vi "WriteToLogFile.vi"(7 "Prepend timestamp":bool, 8 "error in (no error)":errorcluster, 10 "Log entry":string, 11 "Byte Stream File in":refnum<file>) -> (0 "error out":errorcluster, 3 "refnum out":refnum<file>)   [LabVIEW 2019, in "SolutionBuilder.lvlib"]
uses:
  SolutionBuilder/SolutionBuilder.lvlib
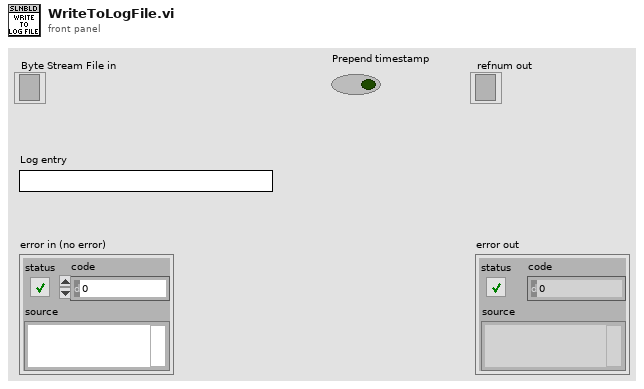
[diagram p1: front panel]
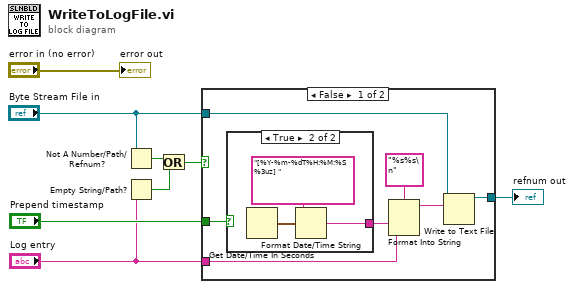
[diagram p0: block diagram]
diagram:
  n1 = Not A Number/Path/Refnum?(number/path/refnum="Byte Stream File in") -> (NaN/Path/Refnum?=w6:bool)
  n2 = Empty String/Path?(string/path="Log entry") -> (empty?=w4:bool)
  n3 = Or(x=w6, y=w4) -> (x .or. y?=w5:bool)
  n4 = case shown="False" w5 {
    tunnel: "Log entry" -> [w13 _]
    tunnel: "Prepend timestamp" -> [w11 _]
    tunnel: "Byte Stream File in" -> [w10 w19]
    tunnel: [w9 w19] -> w1
    frame False {
      n5 = case shown="True" w11 {
        tunnel: [_ w16] -> w15
        frame False {
        }
        frame True {
          n6 = Get Date/Time In Seconds() -> (seconds since 1Jan1904=w17:timestamp)
          n7 = Format Date/Time String(time format string (%c)="[%Y-%m-%dT%H:%M:%S%3uz] ", seconds (now)=w17) -> (date/time string=w16:string)  [unwired: 1 in]
        }
      }
      n8 = Format Into String(format string="%s%s\n", w15, w13) -> (resulting string=w12:string)  [unwired: 2 in, 1 out]
      n9 = Write to Text File(file (use dialog)=w10, text=w12) -> (refnum out=w9:refnum<file>)  [unwired: 2 in, 2 out]
    }
    frame True {
    }
  }
  "refnum out" <- w1
  "error out" <- "error in (no error)"
